vi "Init Hardware.vi"(8 "error in (no error)":errorcluster, 11 "Ocean Optics Driver in":refnum<class "Ocean Optics Driver.lvclass">) -> (0 "error out":errorcluster, 3 "Ocean Optics Driver out":refnum<class "Ocean Optics Driver.lvclass">)   [LabVIEW 2016, in "Ocean Optics Driver.lvclass"]
uses:
  Ocean Optics Driver.lvclass
  C:/GitHub/NHMFL_Core/Libraries/Instruments/VISA Instrument/VISA Instrument.lvclass
  C:/GitHub/NHMFL_Core/Libraries/Instruments/Spectrometer Driver/Spectrometer Driver.lvclass
  VISA Instrument/VISA Instrument.lvclass/VISA Instrument.ctl
  Spectrometer Driver/Spectrometer Driver.lvclass/Spectrometer Driver.ctl
  VISA Instrument/Read VISA resource.vi
  VISA Instrument/Write VISA resource.vi
  Spectrometer Driver/Write Wavelengths.vi
  Read Ocean optics configuration.vi
  <instrlib>/Ocean Optics 2000 4000/Ocean Optics 2000 4000.lvlib
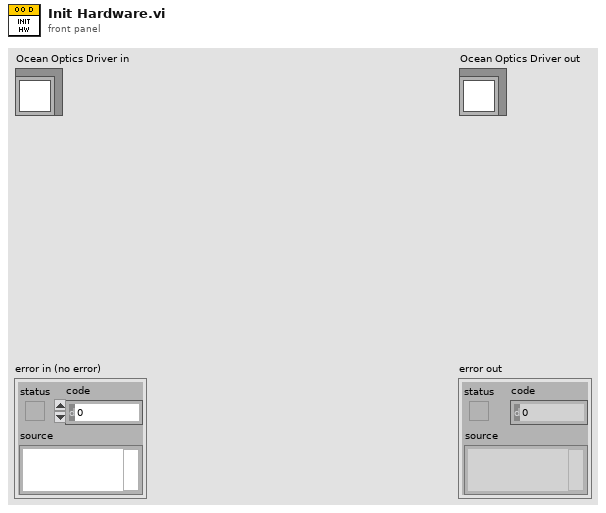
[diagram p1: front panel]
types:
  T1 = typedef "Ruby Spectra.lvclass/Ocean optics configuration.ctl" = cluster{"Integration time":dbl, "Fit parameters":T2, "Fit":bool, "Auto-update params":bool, "Save spectra":bool, "Reference wavelengh":dbl, "Background":path}
  T2 = typedef "Multi-peak Parameters.ctl" = cluster{"Function":enum16{"Gauss", "Lorentz"}, "Window width":dbl, "Initial guess":T3}
  T3 = typedef "Peak Parameters.ctl" = cluster{"Amplitude":dbl, "Center":dbl, "Width":dbl}
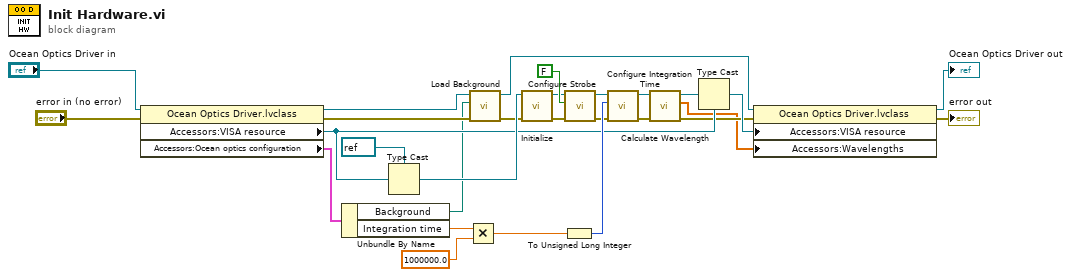
[diagram p0: block diagram]
diagram:
  n1 = property class="Ocean Optics Driver.lvclass"(reference="Ocean Optics Driver in", error in="error in (no error)") -> (reference out=w5:refnum<class "Ocean Optics Driver.lvclass">, error out=w3:errorcluster, "Accessors:VISA resource"=w11:refnum<visa-resource-name>, "Accessors:Ocean optics configuration"=w27:T1)
  n2 = Unbundle By Name(w27) -> ("Background"=w1:path, "Integration time"=w14:dbl)
  n3 = Type Cast(type=refnum<visa-resource-name> refnum ("VISA resource name"), x=w11) -> (*(type *) &x=w25:refnum<visa-resource-name>)
  n4 = Multiply(x=w14, y=1000000.0) -> (x*y=w22:dbl)
  n5 = call-dynamic "Load Background.vi"("error in (no error)"=w3, "Background"=w1, "Ocean Optics Driver in"=w5) -> ("error out"=w2:errorcluster, "Ocean Optics Driver out"=w4:refnum<class "Ocean Optics Driver.lvclass">)  [unwired: 7 in]
  n6 = call <instrlib>:"Initialize.vi"("error in (no error)"=w2, "VISA resource name"=w25) -> ("error out"=w15:errorcluster, "VISA resource name out"=w16:refnum<visa-resource-name>)  [unwired: 1 in, 7 out]
  n7 = To Unsigned Long Integer(number=w22) -> (unsigned 32bit integer=w23:u32)
  n8 = call <instrlib>:"Configure Strobe.vi"("error in (no error)"=w15, "Enable Strobe (Disabled)"=FALSE, "VISA resource name"=w16) -> ("error out"=w18:errorcluster, "VISA resource name out"=w17:refnum<visa-resource-name>)  [unwired: 7 out]
  n9 = call <instrlib>:"Configure Integration Time.vi"("error in (no error)"=w18, "Integration Time (6000)"=w23, "VISA resource name"=w17) -> ("error out"=w19:errorcluster, "VISA resource name out"=w20:refnum<visa-resource-name>)  [unwired: 7 in]
  n10 = call <instrlib>:"Calculate Wavelength.vi"("error in (no error)"=w19, "VISA resource name"=w20) -> ("error out"=w9:errorcluster, "Wavelength (nm)"=w6:dbl[], "VISA resource name out"=w12:refnum<visa-resource-name>)  [unwired: 1 in, 6 out]
  n11 = Type Cast(type=w11, x=w12) -> (*(type *) &x=w10:refnum<visa-resource-name>)
  n12 = property class="Ocean Optics Driver.lvclass"(reference=w4, error in=w9, "Accessors:VISA resource"=w10, "Accessors:Wavelengths"=w6) -> (reference out=→"Ocean Optics Driver out":refnum<class "Ocean Optics Driver.lvclass">, error out=→"error out":errorcluster)
